vi "LVClass_Image get image data U32.vi"(0 "Image in":refnum<class "Image.lvclass">, 5 "Image data":u32[][](array[numeric]), 11 "error in (no error)":errorcluster) -> (4 "Image out":refnum<class "Image.lvclass">, 6 "Image data out":u32[][](array[numeric]), 15 "error out":errorcluster)   [LabVIEW 2020, in "Image.lvclass"]
doc: "Get pixels buffer from 32-bit Image.\n\n--------------------------------------------------------------------------------\n\n<B>ImageIn </B> : Image object.\n<B>ImageOut </B> : Image object.\n<B>buffer </B> : Pixel buffer.\n<B>ErrorIn </B> : Error\n<B>ErrorOut </B> : Error\n\n--------------------------------------------------------------------------------"
uses:
  Image.lvclass
  Image.lvclass/Image.ctl
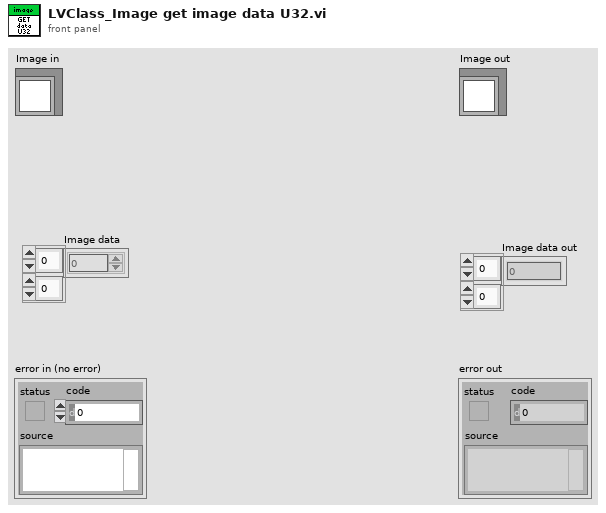
[diagram p1: front panel]
types:
  T1 = typedef "ClassID.ctl" = i64
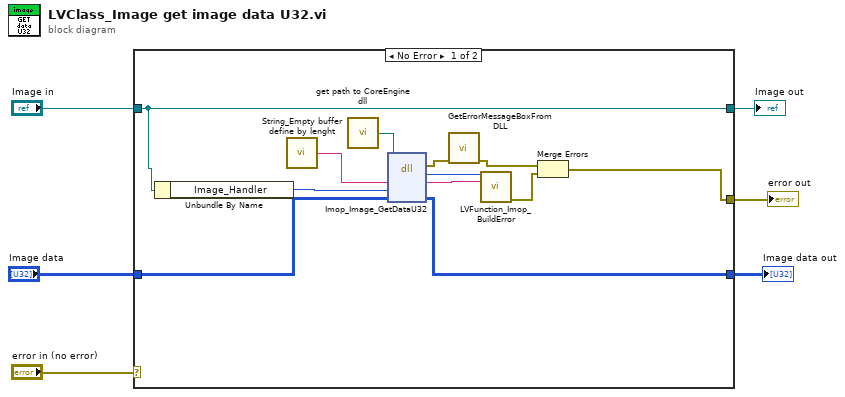
[diagram p0: block diagram]
diagram:
  n1 = case shown="No Error" "error in (no error)" {
    selector: "error in (no error)" -> [_ w21]
    tunnel: [w7 w21] -> w5
    tunnel: [w11 w20] -> w3
    tunnel: "Image in" -> [w11 w20]
    tunnel: "Image data" -> [w15 w19]
    tunnel: [w14 w19] -> w1
    frame No Error {
      n2 = Unbundle By Name(w11) -> ("Image_Handler"=w10:T1)
      n3 = call "String_Empty buffer define by lenght.vi"() -> ("Empty buffer"=w18:string)  [unwired: 1 in]
      n4 = call "get path to CoreEngine dll.vi"() -> ("path to wavekit library"=w13:path)  [unwired: 14 in, 1 out]
      n5 = dll-call lib="D:/soft/HASO_v3/SVN_trunk/ImOpCoreEngine4_LV2011/DLLs/c_interface_vc100.dll" fn="Imop_Image_GetDataU32"(path in=w13, "message"=w18, "Image compat"=w10, "Image data"=w15) -> (error out=w12:errorcluster, "return type"=w17:i32, "message"=w16:string, "Image data"=w14:u32[][])  [unwired: 3 in, 1 out]
      n6 = call "GetErrorMessageBoxFromDLL.vi"("error IN"=w12) -> ("error OUT"=w9:errorcluster)  [unwired: 10 in]
      n7 = call "LVFunction_Imop_BuildError.vi"("code"=w17, "String to Prepend to source (\"\")"=w16) -> ("error out"=w8:errorcluster)  [unwired: 13 in]
      n8 = Merge Errors(w9, w8) -> (w7:errorcluster)
    }
    frame Error {
    }
  }
  "error out" <- w5
  "Image out" <- w3
  "Image data out" <- w1
